vi "Splid RDRr Cluster.vi"(7 "Periodic data":T3, 11 "Error in":errorcluster) -> (1 "Common TS.V":dbl=nan caption="Topside Voltage\nVAC" format="%-1.1f", 2 "Common Wire.R":dbl=nan caption="Wire Resitance\nohm" format="%-1.1f", 3 "Common Wire.I":dbl=nan caption="Supply Current\nAAC" format="%-1.1f", 4 "Connected Indicator PSU":T2 caption="PSU", 6 "Connected Indicator PPC PC Cont":T1 caption="PC", 8 "Connected Indicator PSU HV On":T1 caption="HV", 10 "Connected Indicator PSU Winch Moving":T1 caption="Moving", 12 "Common Wire.Len":dbl=nan caption="Wire Length\nm", 13 "Common Wire.Speed":dbl=nan caption="Wire Speed\nm/s" format="%.2f", 14 "Common Wire.Tension":dbl=nan caption="Wire Tension" format="%.2f", 15 "error out":errorcluster)   [LabVIEW 2011]
uses:
  PCP return data types/RDd return.ctl
  PCP return data types/RA return Analog I.ctl
  PCP return data types/RP return digital IO.ctl
  Connected Satus Bool.ctl
  Active Status Bool.ctl
  Application Structure/Options/Action GFV Settings.ctl
  Application Structure/Options/Options PageID.ctl
panel:
  out "AI.PCP Motor voltage, head voltage (AI 3)":dbl
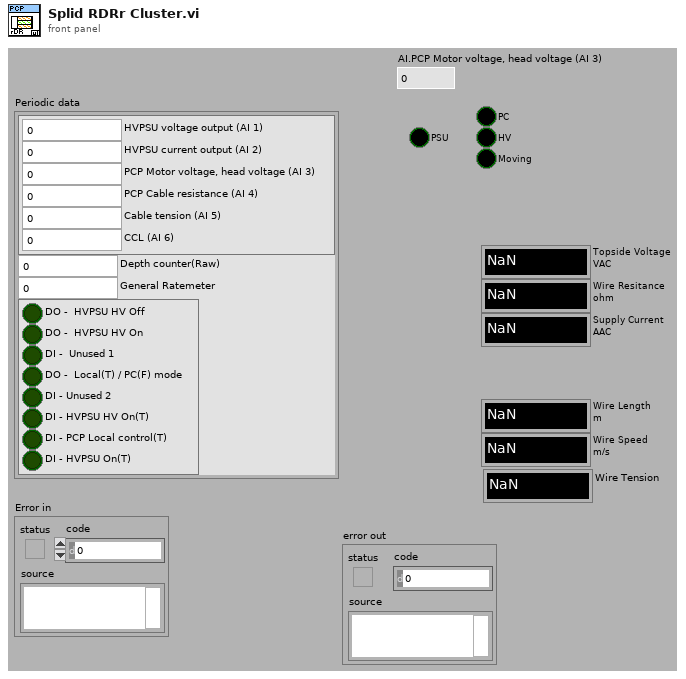
[diagram p1: front panel]
types:
  T1 = typedef "Active Status Bool.ctl" = bool
  T2 = typedef "Connected Satus Bool.ctl" = bool
  T3 = typedef "RDd return.ctl" = cluster{"AI":T4, "Depth counter(Raw)":i32, "General Ratemeter":dbl, "Digital ports":T5}
  T4 = typedef "RA return Analog I.ctl" = cluster{"HVPSU voltage output (AI 1)":dbl, "HVPSU current output (AI 2)":dbl, "PCP Motor voltage, head voltage (AI 3)":dbl, "PCP Cable resistance (AI 4)":dbl, "Cable tension (AI 5)":dbl, "CCL (AI 6)":dbl}
  T5 = typedef "RP return digital IO.ctl" = cluster{"DO -  HVPSU HV Off":bool, "DO -  HVPSU HV On":bool, "DI -  Unused 1":bool, "DO -  Local(T) / PC(F) mode":bool, "DI - Unused 2":bool, "DI - HVPSU HV On(T)":bool, "DI - PCP Local control(T)":bool, "DI - HVPSU On(T)":bool}
  T6 = typedef "Options  All pages and custom.ctl" = cluster{"P 1 (App)":T7, "P 2":T8, "P 3":T9, "P 4":T12, "P 5":T17, "P 6 (Err)":T18, "P 7 (Expert)":T19, "P 8 (Depth)":T21, "C 1":T22, "C 2":T23}
  T7 = typedef "Options Page 1 (App).ctl" = cluster{"Result files":path, "PCP Interface":string, "Tractor/Stroker Interface":string, "Tractor Interface":string, "Modem Status Interface":string, "Audible Alarm":bool, "Force alarm on Technical":bool, "Force alarm on HH":bool, "Force alarm on LL":bool, "Force alarm on H":bool, "Force alarm on L":bool}
  T8 = typedef "Options Page 2.ctl" = cluster{"Solenoid & Relay latching time":u16, "Tractor relay 1":dbl, "Tractor relay 2":dbl, "Tractor Solenoid limit":dbl}
  T9 = typedef "Options Page 3.ctl" = cluster{"Min resistance":dbl, "Max resistance":dbl, "Head voltage range":T10, "Max voltage jump":dbl, "Maximum resistance change":dbl, "Start Telemetry Voltage":dbl, "Start Telemetry Timeout":dbl, "Start Motor Voltage":dbl, "Stop Motor Voltage":dbl, "Pass Mode Warning Voltage":dbl, "Relay Switch Voltage":dbl, "Relay Status Loss Voltage":dbl, "Samples to average":i32, "PSU type DO NOT USE":T11, "Magna OVP":dbl, "Magna Current Limit":dbl}
  T10 = typedef "PCP type List.ctl" = enum16{"0 - 350V", "0 - 450V", "0 - 600V"}
  T11 = typedef "PSU Type.ctl" = enum16{"Unipower", "Magna 8.3A", "Magna 12A", "None"}
  T12 = typedef "Options Page 4.ctl" = cluster{"Solenoid & Relay latching time":u16, "Stroker relay 1":dbl, "Stroker Relay 2":dbl, "Stroker Solenoid limit":dbl, "Force det.":T13, "Stroke force lim.":dbl, "Anchor Enabled Pressure":dbl, "Tacometer puls":dbl, "Default anchor behavior":T14, "Default stroker behavior":T15, "Default stroker force limit (tonne)":dbl, "Slips Size":T16}
  T13 = typedef "Stroke force selector.ctl" = enum16{"Stroke in = node 1", "Strok out = node 1"}
  T14 = typedef "Default anchor behavior.ctl" = enum16{"Do nothing", "Set Anchor", "Release Anchor"}
  T15 = typedef "Default stroker behavior.ctl" = enum16{"Do nothing", "Stop", "Go Out", "Go In"}
  T16 = typedef "Slips Type Radio.ctl" = enum32{"No Selection", "338 MRS", "3,9 MRS"}
  T17 = typedef "Options Page 5.ctl" = cluster{"Solenoid & Relay latching time":u16, "Driller relay 1":dbl, "Driller Relay 2":dbl, "Driller  Solenoid limit":dbl}
  T18 = typedef "Options Page 6 (Err).ctl" = cluster{"Error and event files":path}
  T19 = typedef "Options Page 7 (Expert).ctl" = cluster{"Show Debug":bool, "Log debug messages":bool, "Additional debug messages":bool, "Start Beagle with Simulator data":bool, "Workshop mode":bool, "Modem baud":u16, "enumCANCOM":bool, "Modem sim":T20, "Telemetry Timeout Disable":i32, "Buffer size":i32, "Upd regular data":bool, "Cable comp":cluster{"VMOD1 Voltage(V)":dbl, "VMOD2 Voltage(V)":dbl}}
  T20 = typedef "Modem simulation setup.ctl" = cluster{"Modem dealay sim":bool, "Sim baud Tx":u16, "Bit Error fraction Tx":dbl, "Sim baud Rx":u16, "Bit Error fraction Rx":dbl}
  T21 = typedef "Options Page 8 (Depth).ctl" = cluster{"Winch Spool Circumference":dbl, "Winch Pulses per Revolution":dbl, "Current Depth":dbl}
  T22 = typedef "Options Custom 1.ctl" = cluster{"Depth Updated":bool, "Depth Offset":dbl}
  T23 = typedef "Options Custom 2.ctl" = cluster{"Placeholder":bool}
  T24 = typedef "Action GFV Settings.ctl" = enum16{"Init", "Get From INI", "Put In INI", "Get Settings", "Get Update Index", "Set Setting"}
  T25 = typedef "Options PageID.ctl" = enum16{"P 1 (App)", "P 2", "P 3", "P 4", "P 5", "P 6 (Err)", "P 7 (Expert)", "P 8", "C 1", "C 2"}
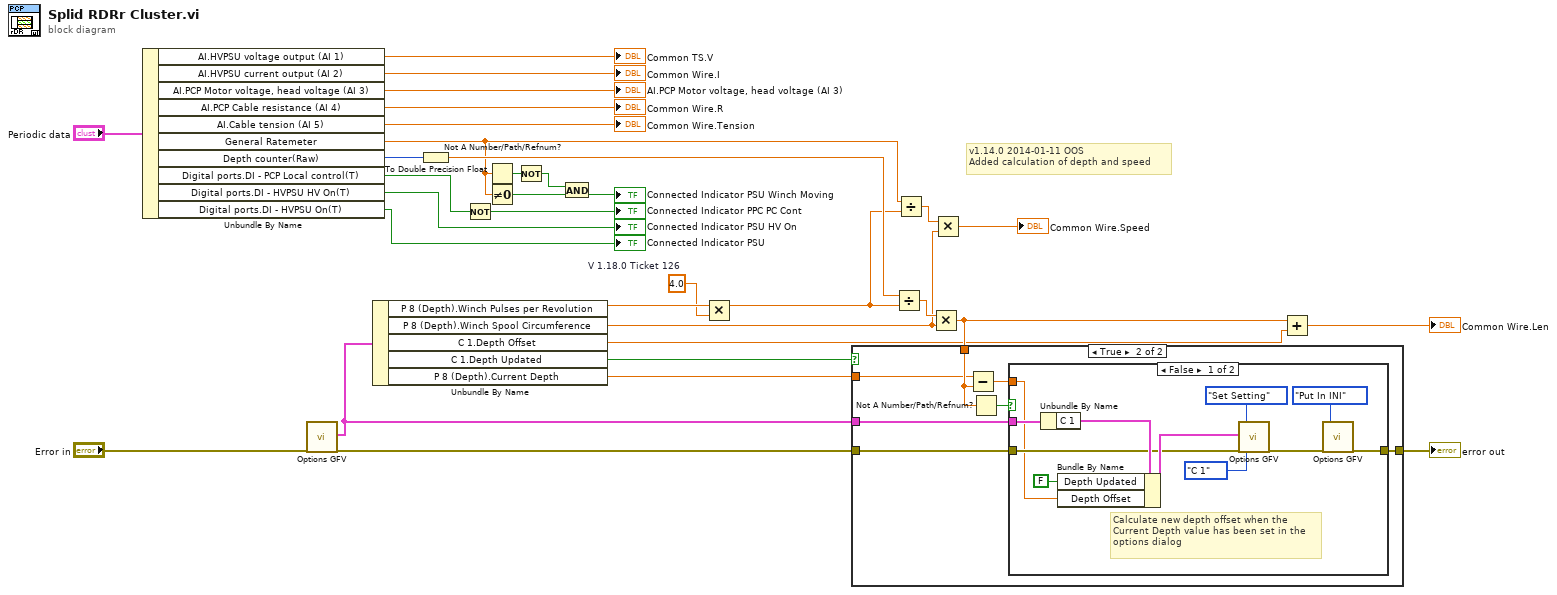
[diagram p0: block diagram]
diagram:
  w1 = 4.0  # V 1.18.0 Ticket 126
  # "v1.14.0 2014-01-11 OOS\nAdded calculation of depth and speed"
  n1 = Unbundle By Name("Periodic data") -> ("AI.HVPSU voltage output (AI 1)"=→"Common TS.V":dbl, "AI.HVPSU current output (AI 2)"=→"Common Wire.I":dbl, "AI.PCP Motor voltage, head voltage (AI 3)"=→"AI.PCP Motor voltage, head voltage (AI 3)":dbl, "AI.PCP Cable resistance (AI 4)"=→"Common Wire.R":dbl, "AI.Cable tension (AI 5)"=→"Common Wire.Tension":dbl, "General Ratemeter"=w14:dbl, "Depth counter(Raw)"=w19:i32, "Digital ports.DI - PCP Local control(T)"=w27:bool, "Digital ports.DI - HVPSU HV On(T)"=→"Connected Indicator PSU HV On":bool, "Digital ports.DI - HVPSU On(T)"=→"Connected Indicator PSU":bool)
  n2 = call "Options GFV.vi"("error in (no error)"="Error in") -> ("Options"=w7:T6, "error out"=w8:errorcluster)  [unwired: 16 in, 1 out]
  n3 = Unbundle By Name(w7) -> ("P 8 (Depth).Winch Pulses per Revolution"=w12:dbl, "P 8 (Depth).Winch Spool Circumference"=w11:dbl, "C 1.Depth Offset"=w4:dbl, "C 1.Depth Updated"=w5:bool, "P 8 (Depth).Current Depth"=w3:dbl)
  n4 = To Double Precision Float(number=w19) -> (double precision float=w17:dbl)
  n5 = Not(x=w27) -> (.not. x?=→"Connected Indicator PPC PC Cont":bool)
  n6 = Not A Number/Path/Refnum?(number/path/refnum=w14) -> (NaN/Path/Refnum?=w22:bool)
  n7 = Not Equal To 0?(x=w14) -> (x != 0?=w28:bool)
  n8 = Not(x=w22) -> (.not. x?=w21:bool)
  n9 = And(x=w21, y=w28) -> (x .and. y?=→"Connected Indicator PSU Winch Moving":bool)
  n10 = Multiply(x=w12, y=w1) -> (x*y=w2:dbl)
  n11 = Divide(x=w17, y=w2) -> (x/y=w16:dbl)
  n12 = Divide(x=w14, y=w2) -> (x/y=w15:dbl)
  n13 = Multiply(x=w16, y=w11) -> (x*y=w6:dbl)
  n14 = case shown="True" w5 {
    tunnel: [w34 w36] -> w9
    tunnel: w8 -> [w34 w37]
    tunnel: w7 -> [_ w38]
    tunnel: w6 -> [_ w41]
    tunnel: w3 -> [_ w40]
    frame False {
    }
    frame True {
      n15 = Subtract(x=w40, y=w41) -> (x-y=w35:dbl)
      n16 = Not A Number/Path/Refnum?(number/path/refnum=w41) -> (NaN/Path/Refnum?=w39:bool)
      n17 = case shown="False" w39 {
        tunnel: w38 -> [w47 _]
        tunnel: w37 -> [w46 w53]
        tunnel: [w42 w53] -> w36
        tunnel: w35 -> [w45 _]
        frame False {
          # "Calculate new depth offset when the\nCurrent Depth value has been set in the\noptions dialog"
          n18 = Unbundle By Name(w47) -> ("C 1"=w50:T22)
          n19 = Bundle By Name(cluster=w50, "Depth Updated"=FALSE ("Placeholder"), "Depth Offset"=w45) -> (w49:T22)
          n20 = call "Options GFV.vi"("Anything"=w49, "error in (no error)"=w46, "Action(Get Settings)"=Action_GFV_Settings."Set Setting", "Setting ID"=Options_PageID."C 1") -> ("error out"=w43:errorcluster)  [unwired: 13 in, 2 out]
          n21 = call "Options GFV.vi"("error in (no error)"=w43, "Action(Get Settings)"=Action_GFV_Settings."Put In INI") -> ("error out"=w42:errorcluster)  [unwired: 15 in, 2 out]
        }
        frame True {
          # "ignore if NaN"
        }
      }
    }
  }
  "error out" <- w9
  n22 = Multiply(x=w15, y=w11) -> (x*y=→"Common Wire.Speed":dbl)
  n23 = Add(x=w6, y=w4) -> (x+y=→"Common Wire.Len":dbl)
